vi "C1--C3.vi"(0 "Starting Position":T5=enum."Far Right", 1 "C1--C3":T4={"1a"=90.0, "2d"=185.0, "2s"=1.0}, 3 "Command Info In":T1, 4 "Switch":string) -> (10 "Command Info Out":T1)   [LabVIEW 2017]
uses:
  <vilib>/Rock Robotics/WPI/Framework/Command Status Info.ctl
  <vilib>/Rock Robotics/WPI/Framework/Completion Status.ctl
  <vilib>/Rock Robotics/WPI/Framework/Completion Notifier.ctl
  Support Code/Starting Position.ctl
  Block Clusters/C1--C3.ctl
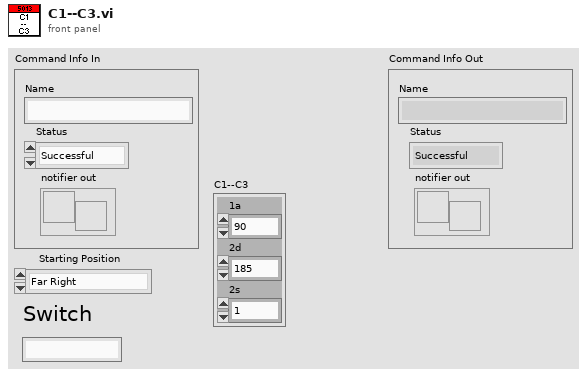
[diagram p1: front panel]
types:
  T1 = typedef "Command Status Info.ctl" = cluster{"Name":string, "Status":T2, "notifier out":T3}
  T2 = typedef "Completion Status.ctl" = enum16{"Successful", "Aborted", "Incomplete"}
  T3 = typedef "Completion Notifier.ctl" = refnum<notifier>
  T4 = typedef "C1--C3.ctl" = cluster{"1a":dbl, "2d":dbl, "2s":dbl}
  T5 = typedef "Starting Position.ctl" = enum16{"Far Left", "Middle", "Far Right"}
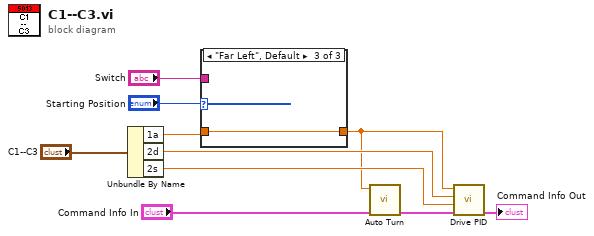
[diagram p0: block diagram]
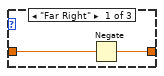
[diagram p2: hidden frame]
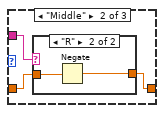
[diagram p3: hidden frame]
diagram:
  n1 = Unbundle By Name("C1--C3") -> ("1a"=w8:dbl, "2d"=w7:dbl, "2s"=w6:dbl)
  n2 = case shown="\"Far Left\", Default" "Starting Position" {
    tunnel: w8 -> [w12 w14 w19]
    tunnel: [w11 w13 w19] -> w3
    tunnel: "Switch" -> [_ w15 _]
    frame "Far Right" {
      n3 = Negate(x=w12) -> (-x=w11:dbl)
    }
    frame "Middle" {
      n4 = case shown="\"R\"" w15 {
        tunnel: w14 -> [w16 w18]
        tunnel: [w16 w17] -> w13
        frame "L", Default {
        }
        frame "R" {
          n5 = Negate(x=w18) -> (-x=w17:dbl)
        }
      }
    }
    frame "Far Left", Default {
    }
  }
  n6 = call "Auto Turn.vi"("Command Info In"="Command Info In", "Target Angle"=w3) -> ("Command Info Out"=w4:T1)  [unwired: 9 in]
  n7 = call "Drive PID.vi"("Command Info In"=w4, "Speed"=w6, "Distance"=w7, "Target Angle"=w3) -> ("Command Info Out"=→"Command Info Out":T1)  [unwired: 7 in]
